vi "Delete Index and Replace Old File.vi"(8 "error in (no error)":errorcluster, 10 "new file path":path, 11 "old file path":path) -> (0 "error out":errorcluster, 3 "new path":path)   [LabVIEW 2023]
doc: "Delete the .index file and replace the original TDMS file with the new one."
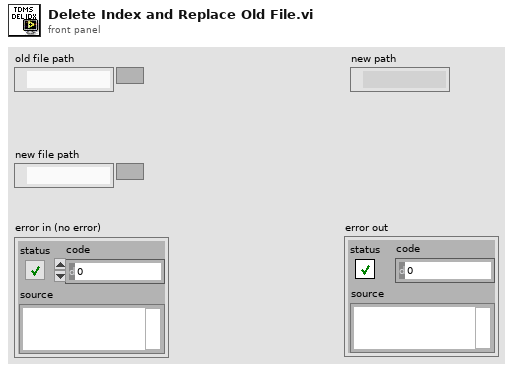
[diagram p1: front panel]
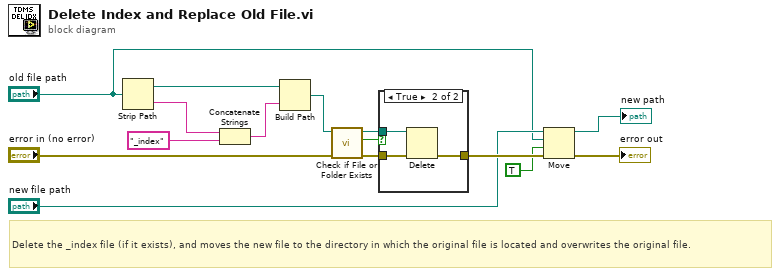
[diagram p0: block diagram]
diagram:
  # "Delete the _index file (if it exists), and moves the new file to the directory in which the original file is located and overwrites the original file."
  n1 = Strip Path(path="old file path") -> (stripped path=w9:path, name=w8:string)
  n2 = Concatenate Strings(w8, "_index" ("string")) -> (w7:string)
  n3 = Build Path(base path=w9, name or relative path=w7) -> (appended path=w3:path)
  n4 = call <vilib>:"Check if File or Folder Exists.vi"("error in (no error)"="error in (no error)", "path"=w3) -> ("error out"=w4:errorcluster, "file or folder exists?"=w1:bool, "dup path"=w2:path)  [unwired: 7 in]
  n5 = case shown="True" w1 {
    tunnel: [w16 w19] -> w15
    tunnel: w4 -> [w16 w18]
    tunnel: w2 -> [_ w17]
    frame False {
    }
    frame True {
      n6 = Delete(path (use dialog)=w17, error in=w18) -> (error out=w19:errorcluster)  [unwired: 3 in, 2 out]
    }
  }
  n7 = Move(source path="new file path", error in=w15, 9:TRUE ("overwrite (F)"), 10:"old file path") -> (error out=→"error out":errorcluster, 3:→"new path":path)  [unwired: 1 in, 1 out]
